vi "AssignAndCount60_2Ch.vi"(7 "Area bits in":bool[](array[boolean])=[FALSE, FALSE, FALSE, FALSE, FALSE, FALSE, FALSE, FALSE, FALSE, FALSE, FALSE, FALSE, FALSE, FALSE, FALSE, FALSE, FALSE, FALSE, FALSE, FALSE, FALSE, FALSE, FALSE, FALSE, FALSE, FALSE, FALSE, FALSE, FALSE, FALSE, FALSE, FALSE, FALSE, FALSE, FALSE, FALSE, FALSE, FALSE, FALSE, FALSE, FALSE, FALSE, FALSE, FALSE, FALSE, FALSE, FALSE, FALSE, FALSE, FALSE, FALSE, FALSE, FALSE, FALSE, FALSE, FALSE, FALSE, FALSE, FALSE, FALSE], 8 "PMT bits Ch2 in":bool[](array[boolean])=[FALSE, FALSE, FALSE, FALSE, FALSE, FALSE, FALSE, FALSE, FALSE, FALSE, FALSE, FALSE, FALSE, FALSE, FALSE, FALSE, FALSE, FALSE, FALSE, FALSE, FALSE, FALSE, FALSE, FALSE, FALSE, FALSE, FALSE, FALSE, FALSE, FALSE, FALSE, FALSE, FALSE, FALSE, FALSE, FALSE, FALSE, FALSE, FALSE, FALSE, FALSE, FALSE, FALSE, FALSE, FALSE, FALSE, FALSE, FALSE, FALSE, FALSE, FALSE, FALSE, FALSE, FALSE, FALSE, FALSE, FALSE, FALSE, FALSE, FALSE], 9 "PMT bits Ch1 in":bool[](array[boolean])=[FALSE, FALSE, FALSE, FALSE, FALSE, FALSE, FALSE, FALSE, FALSE, FALSE, FALSE, FALSE, FALSE, FALSE, FALSE, FALSE, FALSE, FALSE, FALSE, FALSE, FALSE, FALSE, FALSE, FALSE, FALSE, FALSE, FALSE, FALSE, FALSE, FALSE, FALSE, FALSE, FALSE, FALSE, FALSE, FALSE, FALSE, FALSE, FALSE, FALSE, FALSE, FALSE, FALSE, FALSE, FALSE, FALSE, FALSE, FALSE, FALSE, FALSE, FALSE, FALSE, FALSE, FALSE, FALSE, FALSE, FALSE, FALSE, FALSE, FALSE], 10 "Photon counters area 2 in":cluster{u16, u16}, 11 "Photon counters area 1 in":cluster{u16, u16}) -> (2 "Photon counters area 2 out":cluster{u16, u16}, 3 "Photon counters area 1 out":cluster{u16, u16})   [LabVIEW 2012]
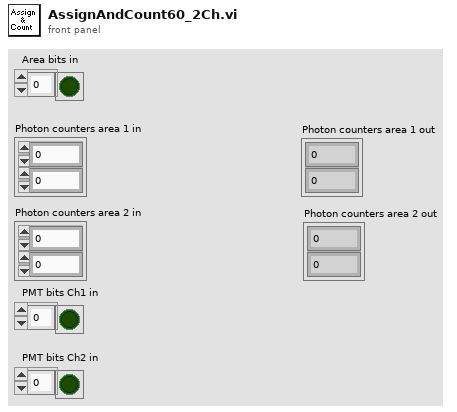
[diagram p1: front panel]
types:
  T1 = cluster{"New high count":u16, "New high count":u16}
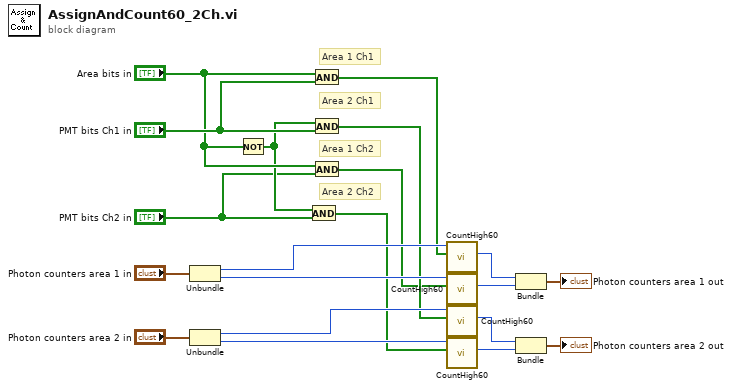
[diagram p0: block diagram]
diagram:
  # "Area 2 Ch2"
  # "Area 1 Ch2"
  # "Area 2 Ch1"
  # "Area 1 Ch1"
  n1 = Unbundle("Photon counters area 1 in") -> (w17:u16, w14:u16)
  n2 = Unbundle("Photon counters area 2 in") -> (w16:u16, w13:u16)
  n3 = Not(x="Area bits in") -> (.not. x?=w4:bool[])
  n4 = And(x=w4, y="PMT bits Ch2 in") -> (x .and. y?=w1:bool[])
  n5 = And(x="Area bits in", y="PMT bits Ch1 in") -> (x .and. y?=w15:bool[])
  n6 = And(x=w4, y="PMT bits Ch1 in") -> (x .and. y?=w6:bool[])
  n7 = And(x="Area bits in", y="PMT bits Ch2 in") -> (x .and. y?=w2:bool[])
  n8 = call "CountHigh60.vi"("60bit input"=w15, "Previous high count"=w17) -> ("New high count"=w12:u16)  [unwired: 9 in]
  n9 = call "CountHigh60.vi"("60bit input"=w2, "Previous high count"=w14) -> ("New high count"=w11:u16)  [unwired: 9 in]
  n10 = call "CountHigh60.vi"("60bit input"=w6, "Previous high count"=w16) -> ("New high count"=w10:u16)  [unwired: 9 in]
  n11 = call "CountHigh60.vi"("60bit input"=w1, "Previous high count"=w13) -> ("New high count"=w9:u16)  [unwired: 9 in]
  n12 = Bundle("New high count"=w12, "New high count"=w11) -> (→"Photon counters area 1 out":T1)  [unwired: 1 in]
  n13 = Bundle("New high count"=w10, "New high count"=w9) -> (→"Photon counters area 2 out":T1)  [unwired: 1 in]
